vi "Get LeafNodes.vi"(8 "error in (no error)":errorcluster caption="错误输入（无错误）", 11 "PanelRootNode 输入":refnum<class "PanelRootNode.lvclass"> caption="DNL_LabVIEW Object in") -> (0 "error out":errorcluster caption="错误输出", 2 "DataNode[]":refnum<data-value>[](array[refnum]), 3 "PanelRootNode 输出":refnum<class "PanelRootNode.lvclass"> caption="DNL_LabVIEW Object out")   [LabVIEW 2016, in "PanelRootNode.lvclass"]
uses:
  PanelRootNode.lvclass
  PanelObject/PanelObject.lvclass
  PanelDataNode/PanelDataNode.lvclass
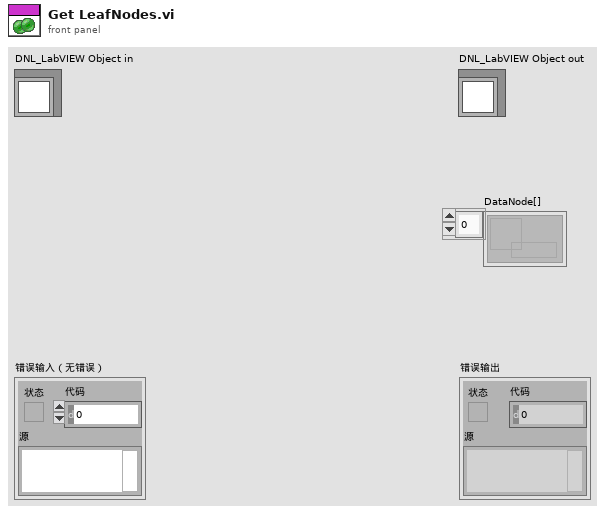
[diagram p1: front panel]
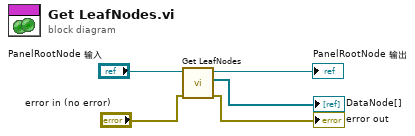
[diagram p0: block diagram]
diagram:
  n1 = call-parent "Get LeafNodes.vi"("error in (no error)"="error in (no error)", "PanelLinkNode 输入"="PanelRootNode 输入") -> ("error out"=→"error out":errorcluster, "DataNode[]"=→"DataNode[]":refnum<data-value>[], "PanelLinkNode 输出"=→"PanelRootNode 输出":refnum<class "PanelRootNode.lvclass">)  [unwired: 7 in]
